vi "C1--SQ Hi.vi"(8 "Command Info In":T2, 10 "C1--S Hi":T1, 11 "Scale":string) -> (0 "Command Info Out":T2)   [LabVIEW 2017]
uses:
  <vilib>/Rock Robotics/WPI/Framework/Command Status Info.ctl
  <vilib>/Rock Robotics/WPI/Framework/Completion Status.ctl
  <vilib>/Rock Robotics/WPI/Framework/Completion Notifier.ctl
  Block Clusters/C1--sq Hi.ctl
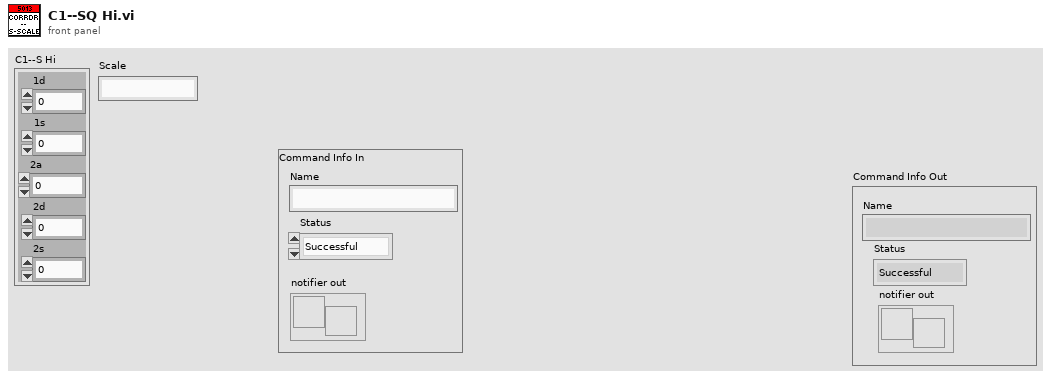
[diagram p1: front panel]
types:
  T1 = typedef "C1--sq Hi.ctl" = cluster{"1d":dbl, "1s":dbl, "2a":dbl, "2d":dbl, "2s":dbl}
  T2 = typedef "Command Status Info.ctl" = cluster{"Name":string, "Status":T3, "notifier out":T4}
  T3 = typedef "Completion Status.ctl" = enum16{"Successful", "Aborted", "Incomplete"}
  T4 = typedef "Completion Notifier.ctl" = refnum<notifier>
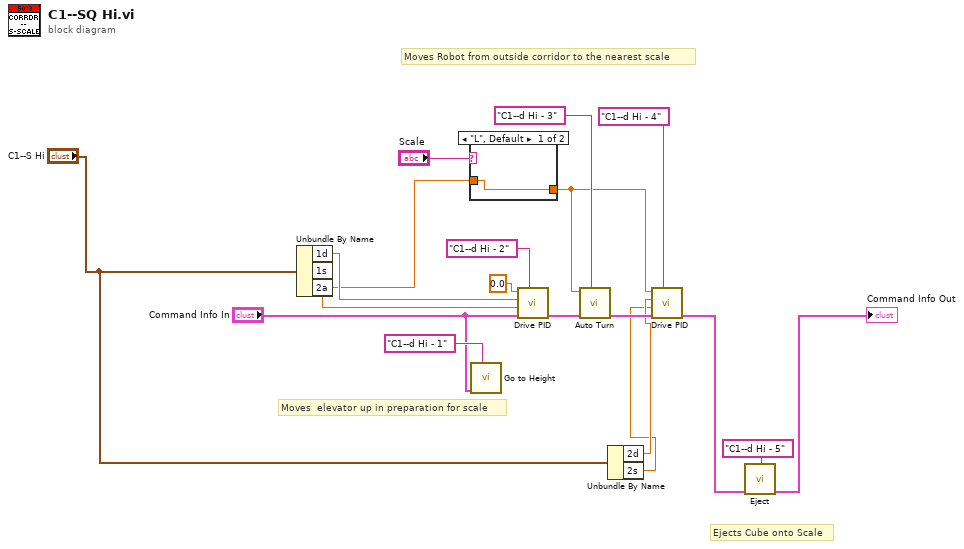
[diagram p0: block diagram]
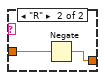
[diagram p2: hidden frame]
diagram:
  # "Ejects Cube onto Scale"
  # "Moves  elevator up in preparation for scale"
  # "Moves Robot from outside corridor to the nearest scale"
  n1 = Unbundle By Name("C1--S Hi") -> ("1d"=w6:dbl, "1s"=w5:dbl, "2a"=w3:dbl)
  n2 = case shown="\"L\", Default" "Scale" {
    tunnel: [w20 w22] -> w8
    tunnel: w3 -> [w20 w21]
    frame "L", Default {
    }
    frame "R" {
      n3 = Negate(x=w21) -> (-x=w22:dbl)
    }
  }
  n4 = call "Go to Height.vi"("Description"="C1--d Hi - 1", "Command Info In"="Command Info In") -> ()  [unwired: 9 in, 1 out]
  n5 = call "Drive PID.vi"("Description"="C1--d Hi - 2", "Command Info In"="Command Info In", "Speed"=w5, "Distance"=w6, "Target Angle"=0.0) -> ("Command Info Out"=w12:T2)  [unwired: 6 in]
  n6 = call "Auto Turn.vi"("Description"="C1--d Hi - 3", "Command Info In"=w12, "Target Angle"=w8) -> ("Command Info Out"=w10:T2)  [unwired: 8 in]
  n7 = Unbundle By Name("C1--S Hi") -> ("2d"=w2:dbl, "2s"=w1:dbl)
  n8 = call "Drive PID.vi"("Description"="C1--d Hi - 4", "Command Info In"=w10, "Speed"=w1, "Distance"=w2, "Target Angle"=w8) -> ("Command Info Out"=w7:T2)  [unwired: 6 in]
  n9 = call "Eject.vi"("Description"="C1--d Hi - 5", "Command Info In"=w7) -> ("Command Info Out"=→"Command Info Out":T2)  [unwired: 9 in]
